vi "Text Definition.vi"(11 "Text in":refnum<class "Text.lvclass">) -> (2 "Definition":T1)   [LabVIEW 2020, in "Conditum.lvlib" / "Columns.lvlib" / "Text.lvclass"]
uses:
  Text.lvclass
  Text.lvclass/Text.ctl
  Definition.ctl
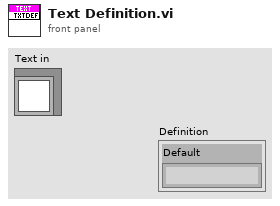
[diagram p1: front panel]
types:
  T1 = typedef "Conditum.lvlib/Columns.lvlib/Text.lvclass/Definition.ctl" = cluster{"Default":string}
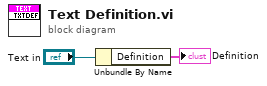
[diagram p0: block diagram]
diagram:
  n1 = Unbundle By Name("Text in") -> ("Definition"=→"Definition":T1)
